vi "数据查询_数据查询.vi"() -> ()   [LabVIEW 2016]
uses:
  <vilib>/Utility/miscctls.llb/LVPointTypeDef.ctl
  <vilib>/Utility/miscctls.llb/LVRowAndColumnUnsignedTypeDef.ctl
  <vilib>/addons/database/_DB Variant To Data/Database Variant To Data.xnode
panel:
  in  "工作模式":string(combo)="全部数据"
  out "连接的字符串":string
  out "选中数据表":string
  in  "查询":bool
  in  "结束日期":string="2020/01/01"
  in  "起始日期":string="2010/01/01"
  out "XY图":cluster{"data":timestamp[], "data":dbl[]}[](graph)
  in  "组合框":string(combo)
  out "数据表":string[][](table)
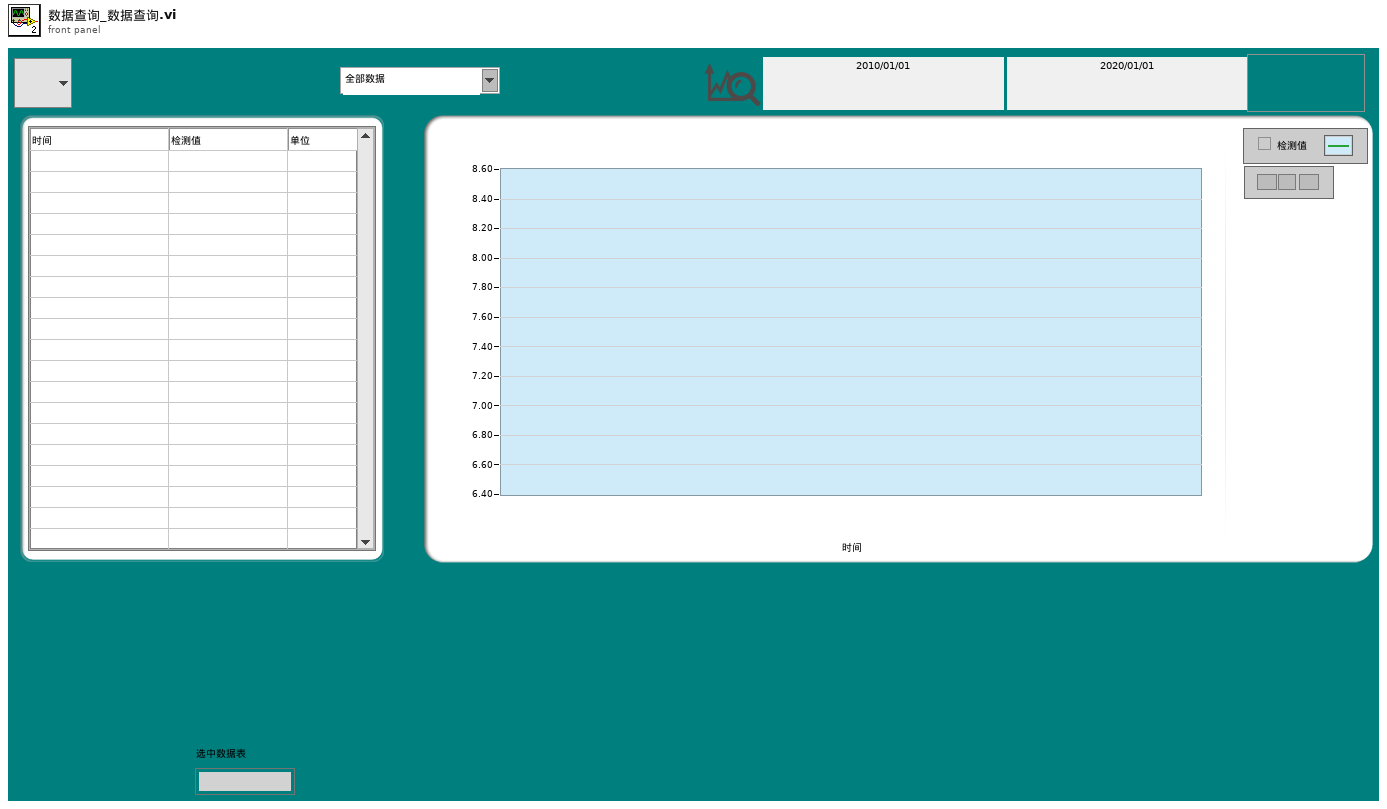
[diagram p1: front panel]
types:
  T1 = typedef "LVPointTypeDef.ctl" = cluster{"Horizontal":i16, "Vertical":i16}
  T2 = typedef "LVRowAndColumnUnsignedTypeDef.ctl" = cluster{"Row":u32, "Column":u32}
  T3 = typedef "LVPoint32TypeDef.ctl" = cluster{"Horizontal":i32, "Vertical":i32}
  T4 = typedef "LVPointDoubleTypeDef.ctl" = cluster{"Cursor X":dbl, "Cursor Y":dbl}
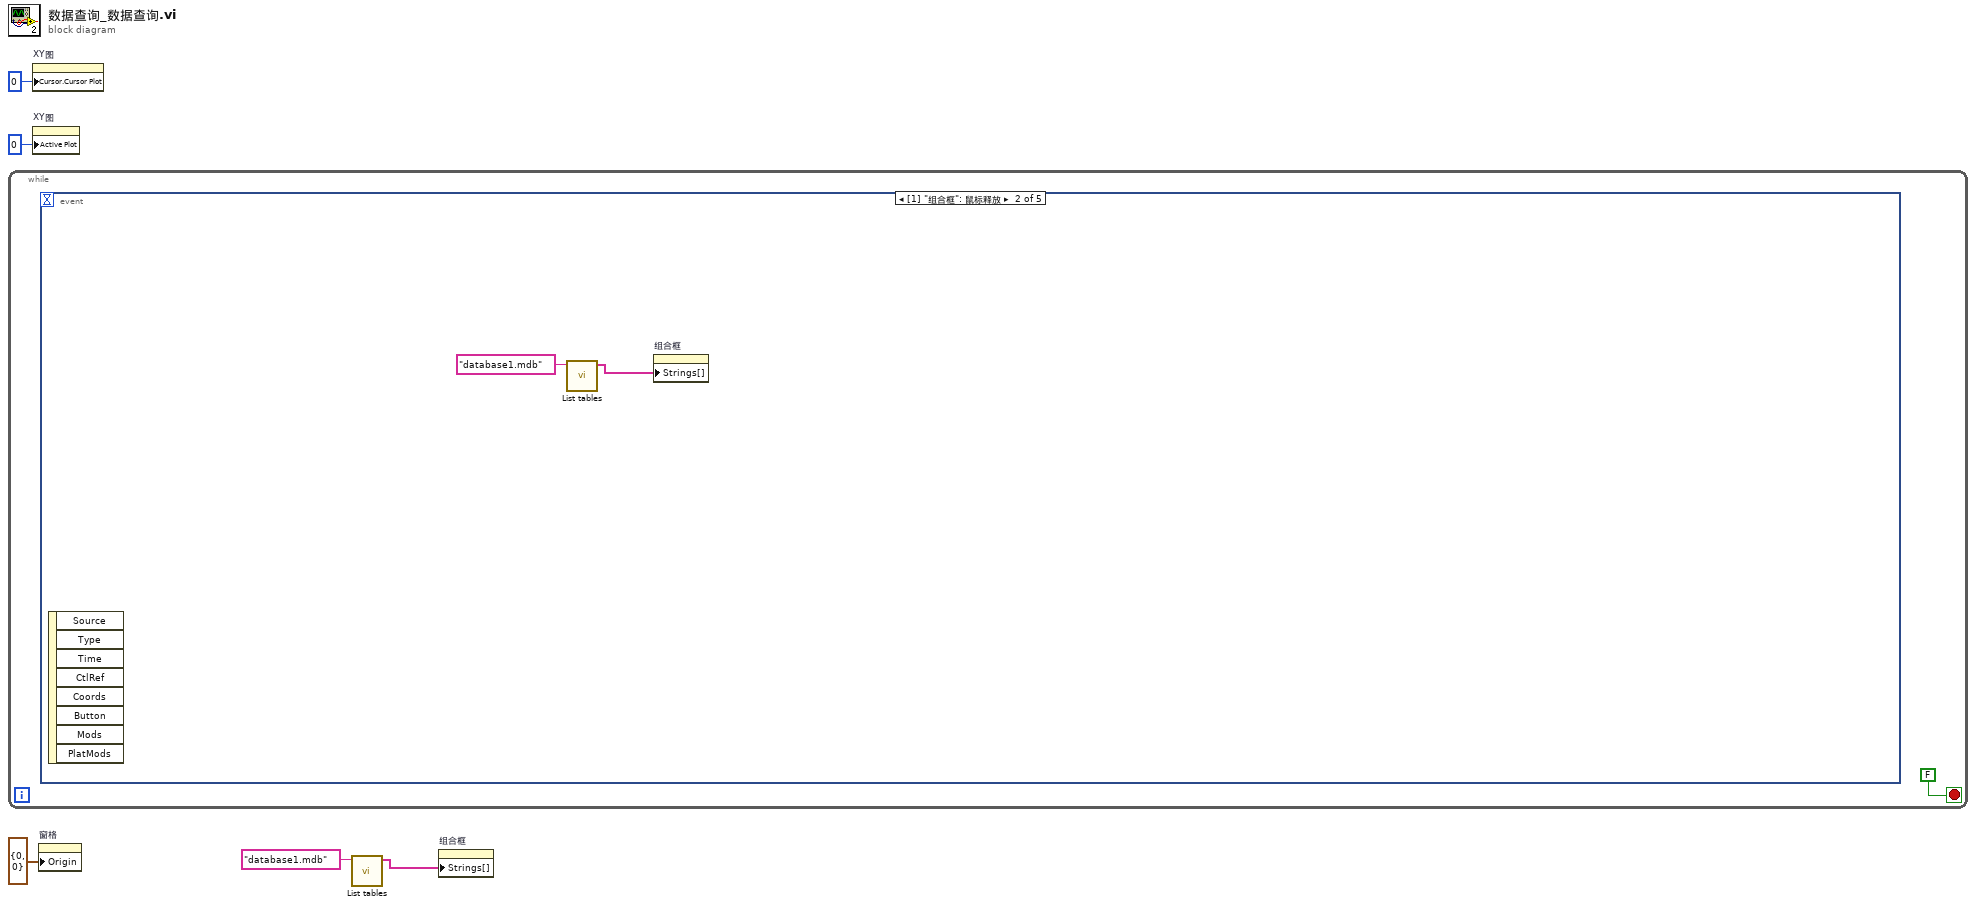
[diagram p0: block diagram]
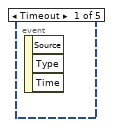
[diagram p2: hidden frame]
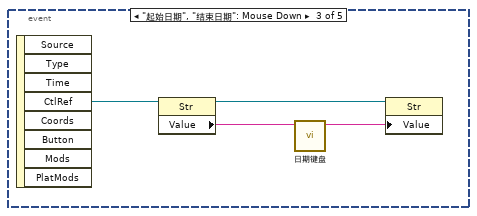
[diagram p3: hidden frame]
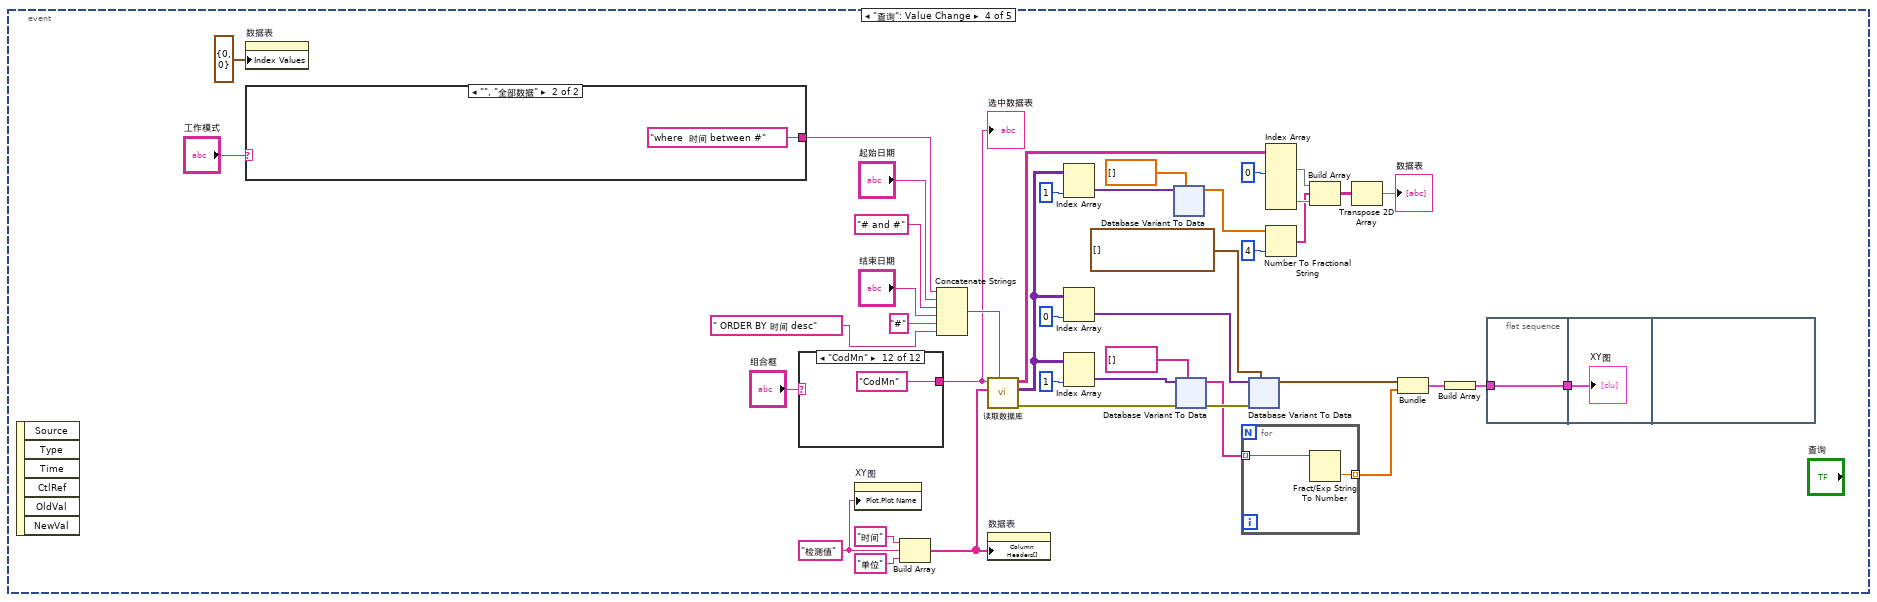
[diagram p4: hidden frame]
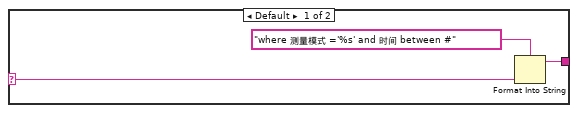
[diagram p5: hidden frame]
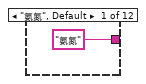
[diagram p6: hidden frame]
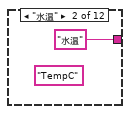
[diagram p7: hidden frame]
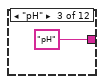
[diagram p8: hidden frame]
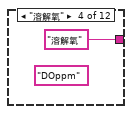
[diagram p9: hidden frame]
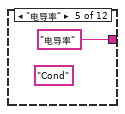
[diagram p10: hidden frame]
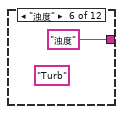
[diagram p11: hidden frame]
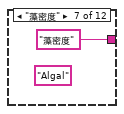
[diagram p12: hidden frame]
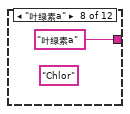
[diagram p13: hidden frame]
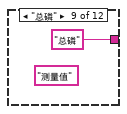
[diagram p14: hidden frame]
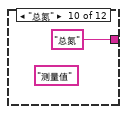
[diagram p15: hidden frame]
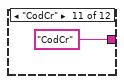
[diagram p16: hidden frame]
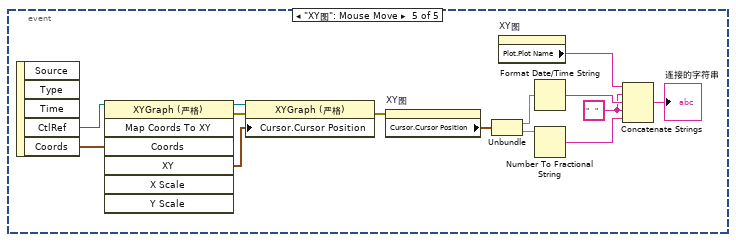
[diagram p17: hidden frame]
diagram:
  n1 = while {
    stop <- FALSE stop-if-true
    n2 = event shown="[1] \"组合框\": 鼠标释放" {
      selector: _ -> [_ _ _ _ _]
      dyn-events: _ -> [_ _ _ _ _]
      timeout: _ -> [_ _ _ _ _]
      event Timeout {
        n3 = event-data() -> ()  [unwired: 1 in, 3 out]
      }
      event "组合框": Mouse Up {
        n4 = event-data() -> ()  [unwired: 1 in, 8 out]
        n5 = call "List tables.vi"("database"="database1.mdb") -> ("tables"=w8:string[])  [unwired: 9 in, 1 out]
        n6 = property on="组合框" class="CmbBox"("Strings[]"=w8) -> ()  [unwired: 2 in, 2 out]
      }
      event "起始日期", "结束日期": Mouse Down {
        n7 = event-data() -> ("CtlRef"=w12:refnum<vi>)  [unwired: 1 in, 7 out]
        n8 = property class="Str"(reference=w12) -> (reference out=w10:refnum<vi>, "Value"=w11:string)  [unwired: 1 in, 1 out]
        n9 = call "日期键盘.vi"("原值"=w11) -> ("x+y"=w9:string)  [unwired: 10 in]
        n10 = property class="Str"(reference=w10, "Value"=w9) -> ()  [unwired: 1 in, 2 out]
      }
      event "查询": Value Change {
        w26 = "检测值"
        n11 = event-data() -> ()  [unwired: 1 in, 6 out]
        n12 = property on="数据表" class="Tbl (严格)"("Index Values"=T2 {"Row"=0, "Column"=0} ("索引值")) -> ()  [unwired: 2 in, 2 out]
        n13 = case shown="\"\", \"全部数据\"" "工作模式" {
          selector: "工作模式" -> [w57 _]
          tunnel: [w55 "where  时间 between #" ("condition")] -> w14
          frame Default {
            n14 = Format Into String(format string="where 测量模式 ='%s' and 时间 between #" ("condition"), w57) -> (resulting string=w55:string)  [unwired: 2 in, 1 out]
          }
          frame "", "全部数据" {
          }
        }
        n15 = case shown="\"CodMn\"" "组合框" {
          tunnel: ["氨氮" "水温" "pH" "溶解氧" "电导率" "浊度" "藻密度" "叶绿素a" "总磷" "总氮" "CodCr" "CodMn"] -> w28
          frame "氨氮", Default {
          }
          frame "水温" {
            (unwired) "TempC"
          }
          frame "pH" {
          }
          frame "溶解氧" {
            (unwired) "DOppm"
          }
          frame "电导率" {
            (unwired) "Cond"
          }
          frame "浊度" {
            (unwired) "Turb"
          }
          frame "藻密度" {
            (unwired) "Algal"
          }
          frame "叶绿素a" {
            (unwired) "Chlor"
          }
          frame "总磷" {
            (unwired) "测量值"
          }
          frame "总氮" {
            (unwired) "测量值"
          }
          frame "CodCr" {
          }
          frame "CodMn" {
          }
        }
        "选中数据表" <- w28
        n16 = property on="XY图" class="XYGraph (严格)"("Plot.Plot Name"=w26) -> ()  [unwired: 2 in, 2 out]
        n17 = Build Array("时间", w26, "单位" ("元素")) -> (w29:string[])
        n18 = Concatenate Strings(w14, "起始日期", "# and #" ("condition"), "结束日期", "#" ("condition"), " ORDER BY 时间 desc" ("字符串")) -> (w53:string)
        n19 = call "读取数据库.vi"("condition"=w53, "显示项"=w29, "组合框"=w28) -> ("error out"=w44:errorcluster, "data"=w23:variant[][], "表格"=w36:string[][])  [unwired: 5 in, 1 out]
        n20 = property on="数据表" class="Tbl (严格)"("Column Headers[]"=w29) -> ()  [unwired: 2 in, 2 out]
        n21 = Index Array(array=w23, index (col)=1 ("禁用的索引 (列)")) -> (element=w21:variant[])  [unwired: 1 in]
        n22 = Index Array(array=w23, index (col)=0 ("禁用的索引 (列)")) -> (element=w47:variant[])  [unwired: 1 in]
        n23 = Index Array(array=w23, index (col)=1 ("禁用的索引 (列)")) -> (element=w45:variant[])  [unwired: 1 in]
        n24 = xnode "Database Variant To Data"("database variant"=w21, "type"=sgl[] []) -> ("data"=w19:sgl[])  [unwired: 1 in, 1 out]
        n25 = xnode "Database Variant To Data"("database variant"=w45, "error in (no error)"=w44, "type"=string[] []) -> ("data"=w27:string[], "error out"=w43:errorcluster)
        n26 = for {
          tunnel: w27 -> [w98] mode=indexing
          tunnel: [w97] -> w13 mode=indexing
          n27 = Fract/Exp String To Number(string=w98) -> (number=w97:dbl)  [unwired: 3 in, 1 out]
        }
        n28 = xnode "Database Variant To Data"("database variant"=w47, "error in (no error)"=w43, "type"=timestamp[] []) -> ("data"=w38:timestamp[])  [unwired: 1 out]
        n29 = Index Array(array=w36, index (col) #1=0 ("禁用的索引 (列)")) -> (element #1=w34:string[], element #3=w24:string[])  [unwired: 5 in, 1 out]
        n30 = Number To Fractional String(number=w19, precision (6)=i16 4 ("精度(6)")) -> (F-format string=w17:string[])  [unwired: 2 in]
        n31 = Build Array(w34, w17, w24) -> (w33:string[][])
        n32 = Transpose 2D Array(2D array=w33) -> (transposed array=→"数据表":string[][])
        n33 = Bundle("data"=w38, w13) -> (w39:cluster{"data":timestamp[], dbl[]})  [unwired: 1 in]
        n34 = Build Array(w39) -> (w40:cluster{"data":timestamp[], dbl[]}[])
        n35 = flat-sequence {
          tunnel: [w111] -> w41
          tunnel: w40 -> [w111]
          tunnel: w41 -> [w112]
          frame #0 {
          }
          frame #1 {
            "XY图" <- w112
          }
          frame #2 {
          }
        }
      }
      event "XY图": Mouse Move {
        w206 = "   " ("字符串")
        n36 = event-data() -> ("CtlRef"=w216:refnum<vi>, "Coords"=w215:T3)  [unwired: 1 in, 3 out]
        n37 = invoke class="XYGraph (严格)" method="Map Coords To XY"(reference=w216, "Coords"=w215) -> (reference out=w214:refnum<vi>, error out=w211:errorcluster, "XY"=w213:cluster{"X":dbl, "Y":dbl})  [unwired: 5 in, 4 out]
        n38 = property class="XYGraph (严格)"(reference=w214, error in=w211, "Cursor.Cursor Position"=w213) -> (error out=w212:errorcluster)  [unwired: 1 out]
        n39 = property on="XY图" class="XYGraph (严格)"(error in=w212) -> ("Cursor.Cursor Position"=w209:T4)  [unwired: 1 in, 2 out]
        n40 = Unbundle(w209) -> ("Cursor X"=w208:dbl, "Cursor Y"=w205:dbl)
        n41 = property on="XY图" class="XYGraph (严格)"() -> ("Plot.Plot Name"=w203:string)  [unwired: 2 in, 2 out]
        n42 = Format Date/Time String(seconds (now)=w208) -> (date/time string=w207:string)  [unwired: 2 in]
        n43 = Number To Fractional String(number=w205) -> (F-format string=w204:string)  [unwired: 3 in]
        n44 = Concatenate Strings(w203, w206, w207, w206, w204) -> (→"连接的字符串":string)
      }
    }
  }
  n45 = property on="XY图" class="XYGraph (严格)"("Cursor.Cursor Plot"=0 ("游标.游标关联曲线")) -> ()  [unwired: 2 in, 2 out]
  n46 = property on="XY图" class="XYGraph (严格)"("Active Plot"=u32 0 ("活动曲线")) -> ()  [unwired: 2 in, 2 out]
  n47 = property on="窗格" class="Pane"("Origin"=T1 {"Horizontal"=0, "Vertical"=0} ("原点")) -> ()  [unwired: 2 in, 2 out]
  n48 = call "List tables.vi"("database"="database1.mdb") -> ("tables"=w1:string[])  [unwired: 9 in, 1 out]
  n49 = property on="组合框" class="CmbBox"("Strings[]"=w1) -> ()  [unwired: 2 in, 2 out]
